vi "MeassurementList.vi"(11 "filenames":string[](array[string])) -> (3 "ListaPomiarów":string[](array[string]))   [LabVIEW 2019]
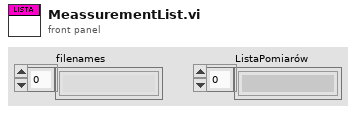
[diagram p1: front panel]
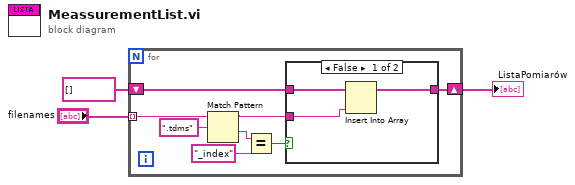
[diagram p0: block diagram]
diagram:
  n1 = for {
    tunnel: "filenames" -> [w11] mode=indexing
    shift-right: [w5] -> w1
    shift-left: string[] [] -> [w6]
    n2 = Match Pattern(string=w11, regular expression=".tdms") -> (before substring=w4:string, after substring=w7:string)  [unwired: 1 in, 2 out]
    n3 = Equal?(x=w7, y="_index") -> (x = y?=w8:bool)
    n4 = case shown="False" w8 {
      tunnel: w4 -> [w12 _]
      tunnel: w6 -> [w14 w15]
      tunnel: [w13 w15] -> w5
      frame False {
        n5 = Insert Into Array(array=w14, new element=w12) -> (w13:string[])  [unwired: 1 in]
      }
      frame True {
      }
    }
  }
  "ListaPomiarów" <- w1
